vi "S2C_Shared_Proc_ErrorCheck.vi"(8 "Error In":errorcluster, 9 "ExpReply?":bool, 10 "Clear Error?":bool, 11 "Reply Text":string) -> (0 "Error Out":errorcluster, 3 "Status":string)   [LabVIEW 2024]
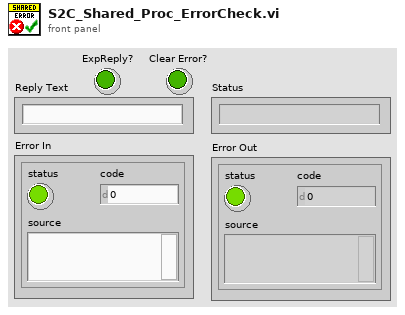
[diagram p1: front panel]
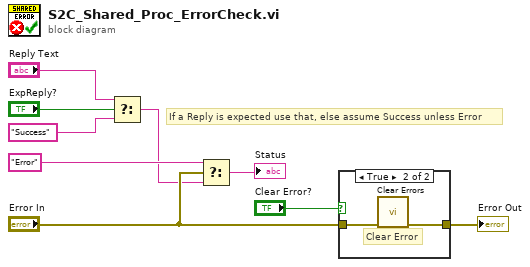
[diagram p0: block diagram]
diagram:
  # "If a Reply is expected use that, else assume Success unless Error"
  n1 = Select(t="Reply Text", s="ExpReply?", f="Success") -> (s? t:f=w1:string)
  n2 = Select(t="Error", s="Error In", f=w1) -> (s? t:f=→"Status":string)
  n3 = case shown="True" "Clear Error?" {
    tunnel: "Error In" -> [w10 w12]
    tunnel: [w10 w11] -> w7
    frame False {
    }
    frame True {
      # "Clear Error"
      n4 = call <vilib>:"Clear Errors.vi"("error in (no error)"=w12) -> ("error out"=w11:errorcluster)  [unwired: 5 in, 1 out]
    }
  }
  "Error Out" <- w7
